vi "Get Time and Date.vi"() -> (3 "Time/Date":string)   [LabVIEW 2019]
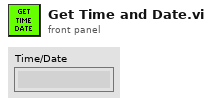
[diagram p1: front panel]
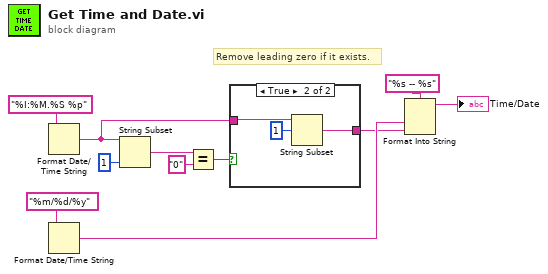
[diagram p0: block diagram]
diagram:
  # "Remove leading zero if it exists."
  n1 = Format Date/Time String(time format string (%c)="%I:%M.%S %p") -> (date/time string=w6:string)  [unwired: 2 in]
  n2 = Format Date/Time String(time format string (%c)="%m/%d/%y") -> (date/time string=w4:string)  [unwired: 2 in]
  n3 = String Subset(string=w6, length (rest)=1 ("length (rest)")) -> (substring=w9:string)  [unwired: 1 in]
  n4 = Equal?(x=w9, y="0") -> (x = y?=w7:bool)
  n5 = case shown="True" w7 {
    tunnel: w6 -> [w12 w15]
    tunnel: [w12 w13] -> w3
    frame False {
    }
    frame True {
      n6 = String Subset(string=w15, offset (0)=1) -> (substring=w13:string)  [unwired: 1 in]
    }
  }
  n7 = Format Into String(format string="%s -- %s", w4, w3) -> (resulting string=→"Time/Date":string)  [unwired: 2 in, 1 out]
